vi "check mapping.vi"(7 "owner":string, 8 "error in":errorcluster, 10 "line":T1, 11 "engine configuration in":refnum<class "engine configuration.lvclass">) -> (0 "error out":errorcluster, 2 "valid?":bool, 3 "engine configuration out":refnum<class "engine configuration.lvclass">)   [LabVIEW 2013, in "Scan Engine editor node.lvclass"]
uses:
  Scan Engine editor node.lvclass
  table line.ctl
  <vilib>/NI/Tag Bus Module Framework/channel/TBM channel.lvclass
  <vilib>/NI/Module Execution Interface/Engine Configuration/engine configuration.lvclass
  <vilib>/NI/Tag Bus/tag/tag descriptor.lvclass/tag descriptor.ctl
  <vilib>/NI/Tag Bus Module Framework/channel/TBM channel.lvclass/TBM channel.ctl
  <vilib>/NI/Module Execution Interface/Engine Configuration/engine configuration.lvclass/engine configuration.ctl
  <vilib>/NI/Tag Bus/tag/read tag name.vi
  <vilib>/NI/Tag Bus Module Framework/channel/Read channel classification.vi
  <vilib>/NI/Tag Bus/tag/tag descriptor.lvclass
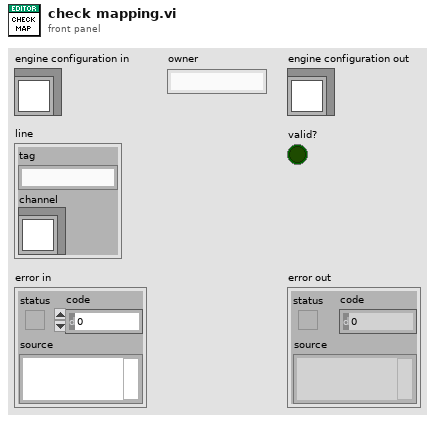
[diagram p1: front panel]
types:
  T1 = typedef "Scan Engine editor node.lvclass/table line.ctl" = cluster{"tag":string, "channel":refnum<class "TBM channel.lvclass">}
  T2 = typedef "TBM channel.lvclass/channel classification.ctl" = enum16{"input data", "output data", "processing parameter", "processing result"}
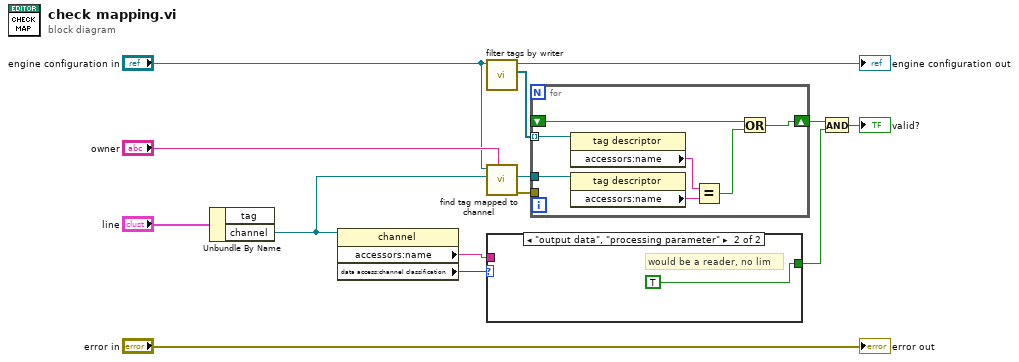
[diagram p0: block diagram]
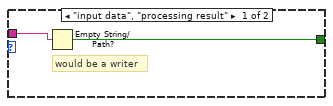
[diagram p2: hidden frame]
diagram:
  n1 = Unbundle By Name("line") -> ("channel"=w12:refnum<class "TBM channel.lvclass">)  [unwired: 1 out]
  n2 = property class="channel"(reference=w12) -> ("accessors:name"=w2:string, "data access:channel classification"=w13:T2)  [unwired: 1 in, 2 out]
  n3 = call <vilib>:"filter tags by writer.vi"("engine configuration in"="engine configuration in") -> ("tag list"=w9:refnum<class "tag descriptor.lvclass">[], "engine configuration out"=→"engine configuration out":refnum<class "engine configuration.lvclass">)  [unwired: 9 in]
  n4 = call <vilib>:"find tag mapped to channel.vi"("owner"="owner", "channel"=w12, "engine configuration in"="engine configuration in") -> ("error out"=w1:errorcluster, "tag"=w8:refnum<class "tag descriptor.lvclass">)  [unwired: 6 in, 1 out]
  n5 = case shown="\"output data\", \"processing parameter\"" w13 {
    tunnel: [w16 TRUE] -> w7
    tunnel: w2 -> [w15 _]
    frame "input data", "processing result" {
      # "would be a writer"
      n6 = Empty String/Path?(string/path=w15) -> (empty?=w16:bool)
    }
    frame "output data", "processing parameter" {
      # "would be a reader, no lim"
    }
  }
  n7 = for {
    tunnel: w9 -> [w24] mode=indexing
    tunnel: w8 -> [w23]
    shift-right: [w18] -> w6
    shift-left: _ -> [w20]
    tunnel: w1 -> [_]
    n8 = property class="tag descriptor"(reference=w24) -> ("accessors:name"=w22:string)  [unwired: 1 in, 2 out]
    n9 = property class="tag descriptor"(reference=w23) -> ("accessors:name"=w21:string)  [unwired: 1 in, 2 out]
    n10 = Equal?(x=w22, y=w21) -> (x = y?=w19:bool)
    n11 = Or(x=w20, y=w19) -> (x .or. y?=w18:bool)
  }
  n12 = And(x=w6, y=w7) -> (x .and. y?=→"valid?":bool)
  "error out" <- "error in"
